vi "solar_ui Unpin.vi"(8 "error in (no error)":errorcluster, 9 "SubPanel":refnum<vi>, 10 "Target":string, 11 "Targets":T1[](array[typedef])) -> (0 "error out":errorcluster, 2 "Target out":string, 3 "VI Refnum":refnum<vi>)   [LabVIEW 2018]
doc: "This unpins (i.e. pops out) the target from the SOLAR user interface."
uses:
  solar_ctl Target Global.ctl
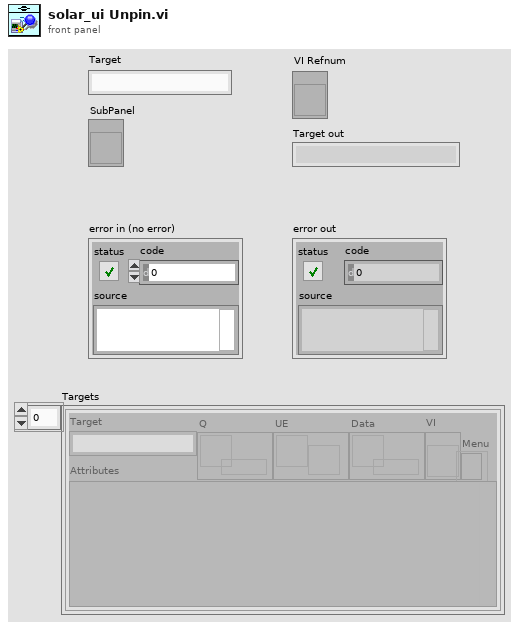
[diagram p1: front panel]
types:
  T1 = typedef "solar_ctl Target Global.ctl" = cluster{"Target":string, "Q":refnum<queue>, "UE":refnum<user-event>, "VI":refnum<vi>, "Menu":refnum<k9>, "Data":refnum<data-value>, "Attributes":variant}
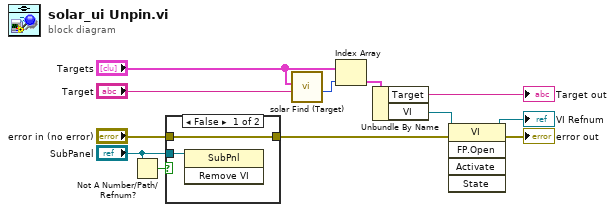
[diagram p0: block diagram]
diagram:
  n1 = Not A Number/Path/Refnum?(number/path/refnum="SubPanel") -> (NaN/Path/Refnum?=w11:bool)
  n2 = case shown="False" w11 {
    tunnel: "SubPanel" -> [w14 _]
    tunnel: [w13 w15] -> w4
    tunnel: "error in (no error)" -> [w13 w15]
    frame False {
      n3 = invoke class="SubPnl" method="Remove VI"(reference=w14) -> ()  [unwired: 2 in, 3 out]
    }
    frame True {
    }
  }
  n4 = call "solar Find (Target).vi"("Target"="Target", "Targets"="Targets") -> ("Target Index"=w6:i32)  [unwired: 8 in, 1 out]
  n5 = Index Array(array="Targets", index=w6) -> (element=w3:T1)
  n6 = Unbundle By Name(w3) -> ("Target"=→"Target out":string, "VI"=w7:refnum<vi>)
  n7 = invoke class="VI" method="FP.Open"(reference=w7, error in=w4) -> (reference out=→"VI Refnum":refnum<vi>, error out=→"error out":errorcluster)  [unwired: 3 in, 3 out]
